vi "Parse Values.vi"(8 "error in":errorcluster, 11 "LV Argument Parser in":refnum<class "LV Argument Parser.lvclass">) -> (0 "error out":errorcluster, 2 "Output":string, 3 "LV Argument Parser out":refnum<class "LV Argument Parser.lvclass">)   [LabVIEW 2023, in "LV ArgParse.lvlib" / "LV Argument Parser.lvclass"]
uses:
  LV Argument Parser.lvclass
  LV Argument Parser.lvclass/LV Argument Parser.ctl
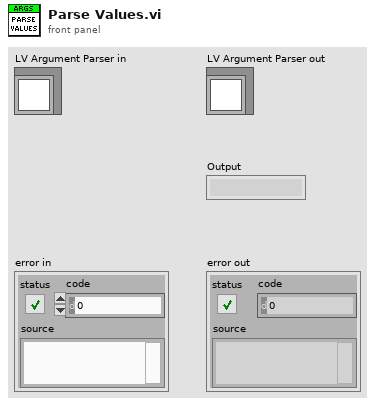
[diagram p1: front panel]
types:
  T1 = enum16{"unknown argument", "invalid argument type", "wrong argument count", "missing required argument"}
  T2 = typedef "LV ArgParse.lvlib/LV Argument Parser.lvclass/Argument Definition.ctl" = cluster{"Name":string, "short (positional)":string, "long (positional)":string, "action":enum16{"store", "store-const", "store-false", "store-true", "append", "append-const", "count", "help", "version"}, "choices":string[], "const":string, "default":string, "dest (=name)":string, "help":string, "Number":i32, "Required":bool, "Type":enum16{"String", "Int", "Uint", "Float", "Bool", "Date", "Path"}}
  T3 = enum16{"store", "store-const", "store-false", "store-true", "append", "append-const", "count", "help", "version"}
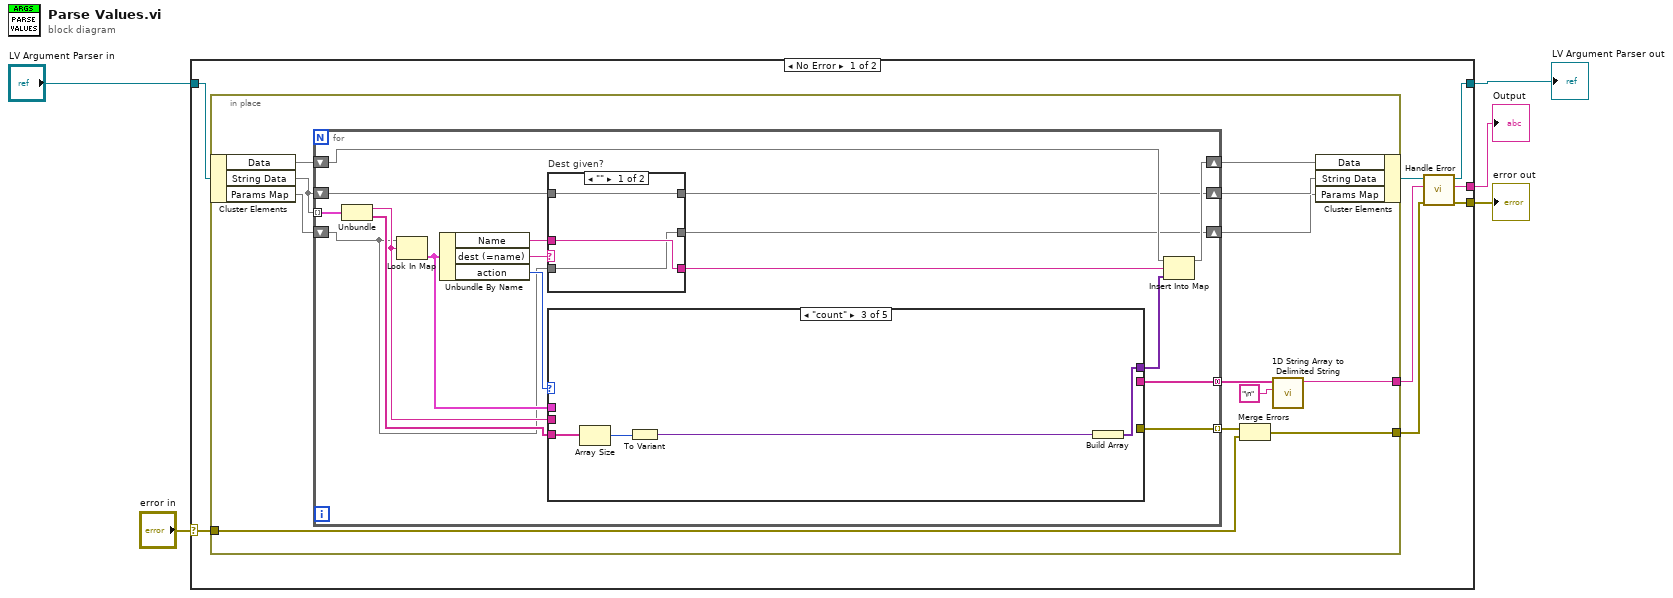
[diagram p0: block diagram]
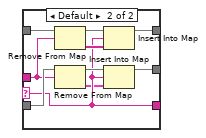
[diagram p2: hidden frame]
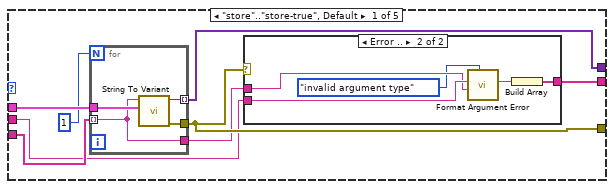
[diagram p3: hidden frame]
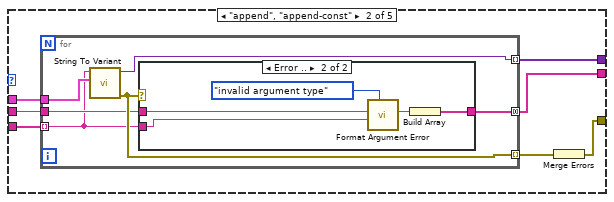
[diagram p5: hidden frame]
diagram:
  n1 = case shown="No Error" "error in" {
    selector: "error in" -> [w8 w96]
    tunnel: [w12 w96] -> w5
    tunnel: "LV Argument Parser in" -> [w13 w95]
    tunnel: [w11 w95] -> w3
    tunnel: [w10 _] -> w1
    frame No Error {
      n2 = in-place {
        in-place-border: w8 -> [w22]
        in-place-border: [w21] -> w7
        in-place-border: [w20] -> w6
        n3 = in-place-cluster #1(w13) -> ("Data"=w19:map{string, variant[]}, "String Data"=w18:map{string, string[]}, "Params Map"=w17:map{string, T2})
        n4 = for {
          tunnel: w18 -> [w42] mode=indexing
          shift-right: [w34] -> w16
          shift-left: w19 -> [w41]
          tunnel: [w39] -> w24 mode=indexing
          tunnel: [w36] -> w25 mode=concatenating
          shift-right: [w31] -> w15
          shift-left: w18 -> [w32]
          shift-right: [w26] -> w14
          shift-left: w17 -> [w27]
          n5 = Unbundle(w42) -> (w33:string, w38:string[])
          n6 = Look In Map(map=w27, key=w33) -> (value=w37:T2)  [unwired: 1 in, 1 out]
          n7 = Unbundle By Name(w37) -> ("Name"=w30:string, "dest (=name)"=w29:string, "action"=w40:T3)
          n8 = case "Dest given?" shown="\"\"" w29 {
            selector: w29 -> [_ w47]
            tunnel: w32 -> [w45 w55]
            tunnel: [w45 w53] -> w31
            tunnel: w30 -> [w44 w48]
            tunnel: [w44 w47] -> w28
            tunnel: w27 -> [w43 w50]
            tunnel: [w43 w49] -> w26
            frame "" {
            }
            frame Default {
              n9 = Remove From Map(10:w48, 11:w55) -> (1:w52:string[], 3:w54:map{string, string[]})  [unwired: 1 out]
              n10 = Remove From Map(10:w48, 11:w50) -> (1:w46:T2, 3:w51:map{string, T2})  [unwired: 1 out]
              n11 = Insert Into Map(map in=w54, key=w47, value=w52) -> (map out=w53:map{string, string[]})  [unwired: 2 out]
              n12 = Insert Into Map(map in=w51, key=w47, value=w46) -> (map out=w49:map{string, T2})  [unwired: 2 out]
            }
          }
          n13 = case shown="\"count\"" w40 {
            tunnel: w38 -> [w62 w79 w94 _ _]
            tunnel: w37 -> [w61 w78 _ _ _]
            tunnel: [w63 w75 w91 _ _] -> w35
            tunnel: [w59 w76 _ _ _] -> w39
            tunnel: w33 -> [w58 w74 _ _ _]
            tunnel: [w56 w73 _ _ _] -> w36
            frame "store".."store-true", Default {
              n14 = for {
                N: 1 -> [_]
                tunnel: [w72] -> w63 mode=indexing
                tunnel: [w71] -> w59
                tunnel: w62 -> [w69] mode=indexing
                tunnel: w61 -> [w70]
                tunnel: [w69] -> w57
                n15 = call "String To Variant.vi"("Type"=w70, "String"=w69) -> ("error out"=w71:errorcluster, "Variant"=w72:variant)  [unwired: 8 in]
              }
              n16 = case shown="Error .." w59 {
                tunnel: w58 -> [_ w68]
                tunnel: w57 -> [_ w67]
                tunnel: [_ w64] -> w56
                frame No Error {
                }
                frame Error {
                  n17 = call "Format Argument Error.vi"("Error Type"=T1."invalid argument type", "Value"=w67, "Name"=w68) -> ("String"=w65:string)  [unwired: 8 in]
                  n18 = Build Array(w65) -> (w64:string[])
                }
              }
            }
            frame "append", "append-const" {
              n19 = for {
                tunnel: w79 -> [w81] mode=indexing
                tunnel: w78 -> [w85]
                tunnel: [w83] -> w77 mode=indexing
                tunnel: [w84] -> w75 mode=indexing
                tunnel: w74 -> [w82]
                tunnel: [w80] -> w73 mode=concatenating
                n20 = call "String To Variant.vi"("Type"=w85, "String"=w81) -> ("error out"=w83:errorcluster, "Variant"=w84:variant)  [unwired: 8 in]
                n21 = case shown="Error .." w83 {
                  tunnel: w82 -> [_ w90]
                  tunnel: w81 -> [_ w89]
                  tunnel: [_ w86] -> w80
                  frame No Error {
                  }
                  frame Error {
                    n22 = call "Format Argument Error.vi"("Error Type"=T1."invalid argument type", "Value"=w89, "Name"=w90) -> ("String"=w87:string)  [unwired: 8 in]
                    n23 = Build Array(w87) -> (w86:string[])
                  }
                }
              }
              n24 = Merge Errors(w77) -> (w76:errorcluster)
            }
            frame "count" {
              n25 = Array Size(array=w94) -> (size(s)=w93:i32)
              n26 = To Variant(anything=w93) -> (Variant=w92:variant)
              n27 = Build Array(w92) -> (w91:variant[])
            }
            frame "help" {
            }
            frame "version" {
            }
          }
          n28 = Insert Into Map(map in=w41, key=w28, value=w35) -> (map out=w34:map{string, variant[]})  [unwired: 2 out]
        }
        n29 = Merge Errors(w24, w22) -> (w20:errorcluster)
        n30 = call <vilib>:"1D String Array to Delimited String.vi"("delimiter"="\n", "string array"=w25) -> ("delimited string"=w21:string)  [unwired: 9 in]
        n31 = in-place-cluster #1("Data"=w16, "String Data"=w15, "Params Map"=w14) -> (w9:refnum<class "LV Argument Parser.lvclass">)
      }
      n32 = call "Handle Error.vi"("error in (no error)"=w6, "delimited string"=w7, "LV Argument Parser in"=w9) -> ("error out"=w12:errorcluster, "Output"=w10:string, "LV Argument Parser out"=w11:refnum<class "LV Argument Parser.lvclass">)  [unwired: 6 in]
    }
    frame Error {
    }
  }
  "error out" <- w5
  "LV Argument Parser out" <- w3
  "Output" <- w1
